vi "Set_Wind_CupSize.vi"(1 "Wind cup size":i16) -> (0 "Succes?":bool)   [LabVIEW 2013]
uses:
  VantagePro.dll
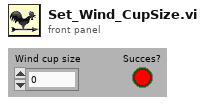
[diagram p1: front panel]
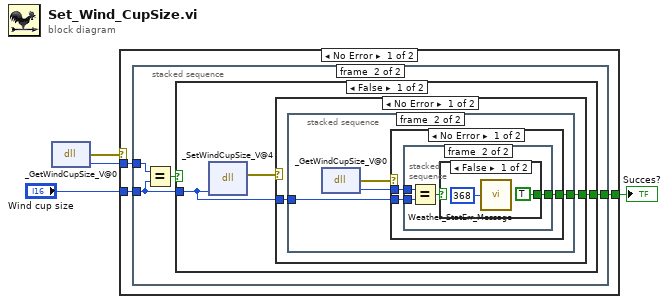
[diagram p0: block diagram]
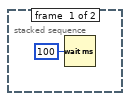
[diagram p2: hidden frame]
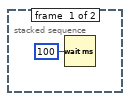
[diagram p3: hidden frame]
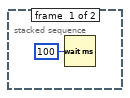
[diagram p4: hidden frame]
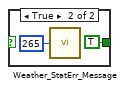
[diagram p5: hidden frame]
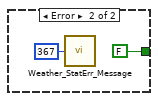
[diagram p6: hidden frame]
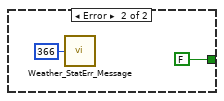
[diagram p7: hidden frame]
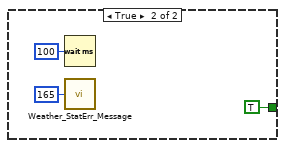
[diagram p8: hidden frame]
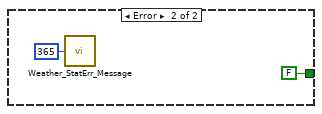
[diagram p9: hidden frame]
diagram:
  n1 = dll-call lib="C:/Users/Bob van Eijk/Desktop/LabView Projects 13/HiSPARC Weather Station/Develop/VantagePro.dll" fn="_GetWindCupSize_V@0" label="Get Wind Cup Size"() -> (error out=w2:errorcluster, "return type"=w1:i16)  [unwired: 3 in, 1 out]
  n2 = case shown="No Error" w2 {
    tunnel: [w7 FALSE] -> w4
    tunnel: "Wind cup size" -> [w6 _]
    tunnel: w1 -> [w5 _]
    frame No Error {
      n3 = stacked-sequence {
        tunnel: [_ w12] -> w7
        tunnel: w6 -> [_ w10]
        tunnel: w5 -> [_ w11]
        frame #0 {
          n4 = Wait (ms)(milliseconds to wait=u32 100) -> ()  [unwired: 1 out]
        }
        frame #1 {
          n5 = Equal?(x=w11, y=w10) -> (x = y?=w9:bool)
          n6 = case shown="False" w9 {
            tunnel: [w15 TRUE] -> w12
            tunnel: w10 -> [w13 _]
            frame False {
              n7 = dll-call lib="C:/Users/Bob van Eijk/Desktop/LabView Projects 13/HiSPARC Weather Station/Develop/VantagePro.dll" fn="_SetWindCupSize_V@4" label="Set Wind Cup Size"("WindCModel"=w13) -> (error out=w14:errorcluster)  [unwired: 4 in, 2 out]
              n8 = case shown="No Error" w14 {
                tunnel: w13 -> [w17 _]
                tunnel: [w16 FALSE] -> w15
                frame No Error {
                  n9 = stacked-sequence {
                    tunnel: w17 -> [_ w22]
                    tunnel: [_ w21] -> w16
                    frame #0 {
                      n10 = Wait (ms)(milliseconds to wait=u32 100) -> ()  [unwired: 1 out]
                    }
                    frame #1 {
                      n11 = dll-call lib="C:/Users/Bob van Eijk/Desktop/LabView Projects 13/HiSPARC Weather Station/Develop/VantagePro.dll" fn="_GetWindCupSize_V@0" label="Get Wind Cup Size"() -> (error out=w19:errorcluster, "return type"=w20:i16)  [unwired: 3 in, 1 out]
                      n12 = case shown="No Error" w19 {
                        tunnel: w22 -> [w25 _]
                        tunnel: [w23 FALSE] -> w21
                        tunnel: w20 -> [w24 _]
                        frame No Error {
                          n13 = stacked-sequence {
                            tunnel: w25 -> [_ w30]
                            tunnel: w24 -> [_ w29]
                            tunnel: [_ w27] -> w23
                            frame #0 {
                              n14 = Wait (ms)(milliseconds to wait=u32 100) -> ()  [unwired: 1 out]
                            }
                            frame #1 {
                              n15 = Equal?(x=w29, y=w30) -> (x = y?=w28:bool)
                              n16 = case shown="False" w28 {
                                tunnel: [TRUE TRUE] -> w27
                                frame False {
                                n17 = call "Weather_StatErr_Message.vi"("Message number"=368) -> ()  [unwired: 1 out]
                                }
                                frame True {
                                n18 = call "Weather_StatErr_Message.vi"("Message number"=265) -> ()  [unwired: 1 out]
                                }
                              }
                            }
                          }
                        }
                        frame Error {
                          n19 = call "Weather_StatErr_Message.vi"("Message number"=367) -> ()  [unwired: 1 out]
                        }
                      }
                    }
                  }
                }
                frame Error {
                  n20 = call "Weather_StatErr_Message.vi"("Message number"=366) -> ()  [unwired: 1 out]
                }
              }
            }
            frame True {
              n21 = Wait (ms)(milliseconds to wait=u32 100) -> ()  [unwired: 1 out]
              n22 = call "Weather_StatErr_Message.vi"("Message number"=165) -> ()  [unwired: 1 out]
            }
          }
        }
      }
    }
    frame Error {
      n23 = call "Weather_StatErr_Message.vi"("Message number"=365) -> ()  [unwired: 1 out]
    }
  }
  "Succes?" <- w4
